vi "Delta robot inverse kinematic for YZ-pane.vi"(4 "re":dbl=224.0 format="%#_13g", 5 "rf":dbl=144.0 format="%#_13g", 6 "e":dbl=39.092 format="%#_13g", 7 "f":dbl=63.127 format="%#_13g", 8 "z0":dbl format="%#_13g", 9 "y0":dbl format="%#_13g", 10 "x0":dbl format="%#_13g") -> (0 "theta":dbl, 1 "non-existing point":bool)   [LabVIEW 2019]
panel:
  out "zj":dbl
  out "yj":dbl
  out "d?":dbl
  out "d":dbl
  out "b":dbl
  out "y0 shift center to edge":dbl
  out "a":dbl
  out "y1":dbl
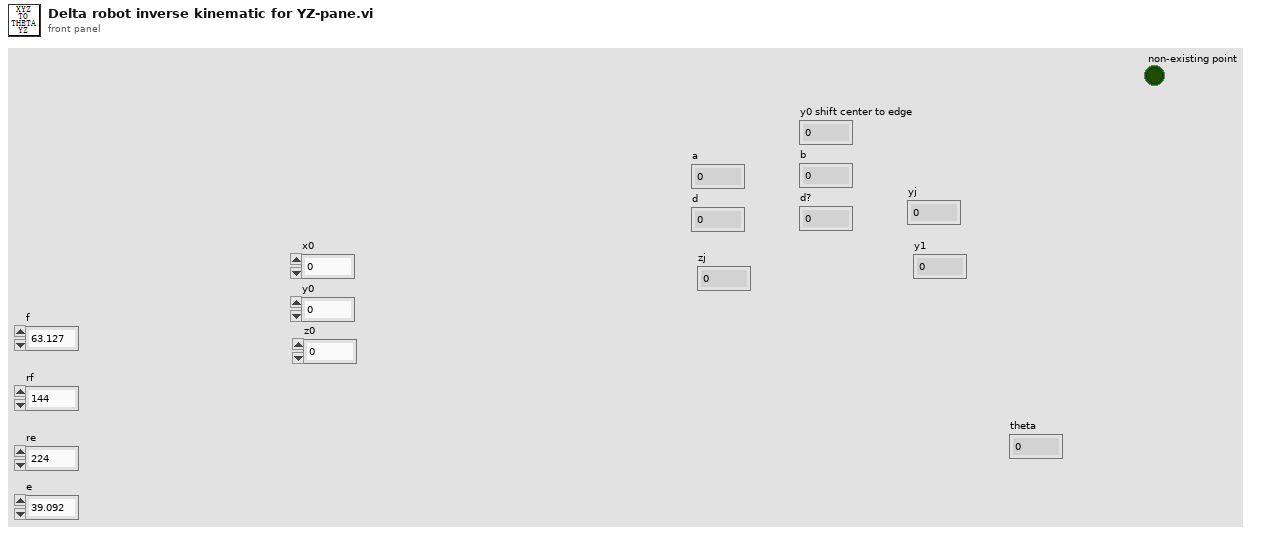
[diagram p1: front panel]
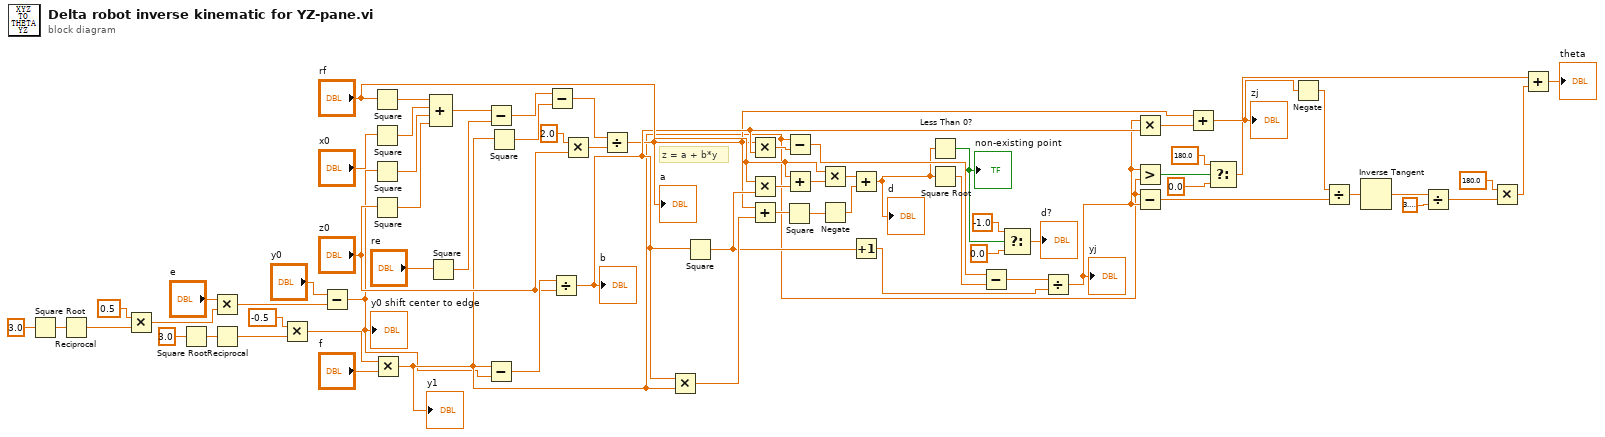
[diagram p0: block diagram]
diagram:
  # "z = a + b*y"
  n1 = Square Root(x=3.0) -> (sqrt(x)=w61:dbl)
  n2 = Reciprocal(x=w61) -> (1/x=w62:dbl)
  n3 = Multiply(x=0.5, y=w62) -> (x*y=w58:dbl)
  n4 = Square Root(x=3.0) -> (sqrt(x)=w64:dbl)
  n5 = Multiply(x="e", y=w58) -> (x*y=w56:dbl)
  n6 = Reciprocal(x=w64) -> (1/x=w63:dbl)
  n7 = Multiply(x=-0.5, y=w63) -> (x*y=w67:dbl)
  n8 = Subtract(x="y0", y=w56) -> (x-y=w4:dbl)
  "y0 shift center to edge" <- w4
  n9 = Square(x="rf") -> (x^2=w51:dbl)
  n10 = Square(x="x0") -> (x^2=w54:dbl)
  n11 = Square(x=w4) -> (x^2=w53:dbl)
  n12 = Square(x="z0") -> (x^2=w52:dbl)
  n13 = Multiply(x=w67, y="f") -> (x*y=w11:dbl)
  "y1" <- w11
  n14 = Square(x="re") -> (x^2=w48:dbl)
  n15 = Compound Arithmetic op=ADD(w51, w54, w53, w52) -> (w50:dbl)
  n16 = Subtract(x=w50, y=w48) -> (x-y=w47:dbl)
  n17 = Subtract(x=w11, y=w4) -> (x-y=w42:dbl)
  n18 = Square(x=w11) -> (x^2=w46:dbl)
  n19 = Subtract(x=w47, y=w46) -> (x-y=w45:dbl)
  n20 = Divide(x=w42, y="z0") -> (x/y=w21:dbl)
  "b" <- w21
  n21 = Multiply(x=2.0, y="z0") -> (x*y=w43:dbl)
  n22 = Divide(x=w45, y=w43) -> (x/y=w19:dbl)
  "a" <- w19
  n23 = Multiply(x=w21, y=w11) -> (x*y=w40:dbl)
  n24 = Square(x=w21) -> (x^2=w23:dbl)
  n25 = Multiply(x=w19, y=w21) -> (x*y=w28:dbl)
  n26 = Multiply(x="rf", y=w23) -> (x*y=w37:dbl)
  n27 = Add(x=w19, y=w40) -> (x+y=w39:dbl)
  n28 = Square(x=w39) -> (x^2=w38:dbl)
  n29 = Subtract(x=w11, y=w28) -> (x-y=w27:dbl)
  n30 = Add(x="rf", y=w37) -> (x+y=w36:dbl)
  n31 = Multiply(x="rf", y=w36) -> (x*y=w33:dbl)
  n32 = Negate(x=w38) -> (-x=w34:dbl)
  n33 = Add(x=w33, y=w34) -> (x+y=w26:dbl)
  "d" <- w26
  n34 = Increment(x=w23) -> (x+1=w22:dbl)
  n35 = Less Than 0?(x=w26) -> (x < 0?=w32:bool)
  "non-existing point" <- w32
  n36 = Square Root(x=w26) -> (sqrt(x)=w25:dbl)
  n37 = Subtract(x=w27, y=w25) -> (x-y=w24:dbl)
  n38 = Select(t=-1.0, s=w32, f=0.0) -> (s? t:f=→"d?":dbl)
  n39 = Divide(x=w24, y=w22) -> (x/y=w12:dbl)
  "yj" <- w12
  n40 = Multiply(x=w12, y=w21) -> (x*y=w20:dbl)
  n41 = Greater?(x=w12, y=w11) -> (0:w10:bool)
  n42 = Subtract(x=w11, y=w12) -> (x-y=w15:dbl)
  n43 = Add(x=w19, y=w20) -> (x+y=w17:dbl)
  "zj" <- w17
  n44 = Select(t=180.0, s=w10, f=0.0) -> (s? t:f=w7:dbl)
  n45 = Negate(x=w17) -> (-x=w16:dbl)
  n46 = Divide(x=w16, y=w15) -> (x/y=w3:dbl)
  n47 = Inverse Tangent(1:w3) -> (0:w2:dbl)
  n48 = Divide(x=w2, y=3.141592653589793) -> (x/y=w1:dbl)
  n49 = Multiply(x=180.0, y=w1) -> (x*y=w13:dbl)
  n50 = Add(x=w7, y=w13) -> (x+y=→"theta":dbl)
